vi "white_out_TC_zone.vi"(8 "error in (no error)":errorcluster, 10 "Blackout?":bool, 11 "Refnum in":T1) -> (0 "error out":errorcluster, 3 "Refnum out":T1)   [LabVIEW 2019]
uses:
  <vilib>/vision/Image Controls.llb/IMAQ Image.ctl
  ParametersGlobal.vi
  <vilib>/vision/NI_Vision_Development_Module.lvlib
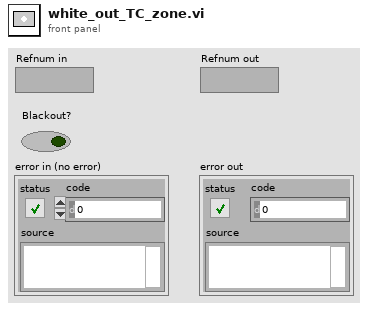
[diagram p1: front panel]
types:
  T1 = typedef "IMAQ Image.ctl" = refnum<image>
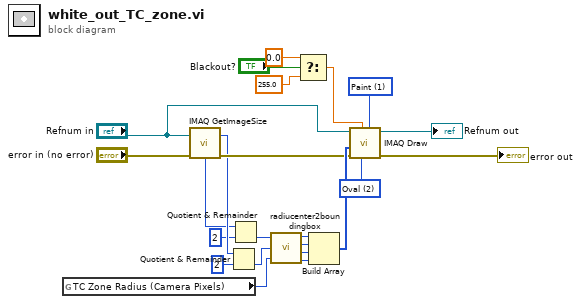
[diagram p0: block diagram]
diagram:
  w21 = u16 1 items=["Frame", "Paint", "Invert Frame", "Invert Paint"] ("Draw Mode")
  w10 = u16 2 items=["Line", "Rectangle", "Oval"] ("Shape to draw")
  n1 = global read "ParametersGlobal.vi" "TC Zone Radius (Camera Pixels)"() -> (w19:i32)
  n2 = call "IMAQ GetImageSize"("Image"="Refnum in", "error in (no error)"="error in (no error)") -> ("Y Resolution"=w8:i32, "X Resolution"=w6:i32, "error out"=w11:errorcluster)  [unwired: 2 in]
  n3 = Quotient & Remainder(x=w8, y=2) -> (floor(x/y)=w18:i32)  [unwired: 1 out]
  n4 = Quotient & Remainder(x=w6, y=2) -> (floor(x/y)=w17:i32)  [unwired: 1 out]
  n5 = call "radiucenter2boundingbox.vi"("Radius"=w19, "ycenter"=w18, "xcenter"=w17) -> ("Bottom"=w16:i32, "Right"=w15:i32, "Top"=w14:i32, "Left"=w13:i32)  [unwired: 2 in]
  n6 = Select(t=0.0, s="Blackout?", f=sgl 255.0 ("Pixel Color")) -> (s? t:f=w1:dbl)
  n7 = Build Array(w13, w14, w15, w16) -> (w20:i32[])
  n8 = call "IMAQ Draw"("Draw Mode"=w21, "Shape to draw"=w10, "Pixel Color"=w1, "error in (no error)"=w11, "Coordinates"=w20, "Image Src"="Refnum in") -> ("error out"=→"error out":errorcluster, "Image Dst Out"=→"Refnum out":T1)  [unwired: 4 in]
